vi "template-name.other.vi"(8 "error in (no error)":errorcluster, 10 "Numeric":dbl, 11 "class template-name in":refnum<class "template-name.lvclass">) -> (0 "error out":errorcluster, 2 "indicator template-name 2":dbl, 3 "class template-name out":refnum<class "template-name.lvclass">)   [LabVIEW 2019, in "template-name.lvclass"]
uses:
  template-name.lvclass
  template-name.control.ctl
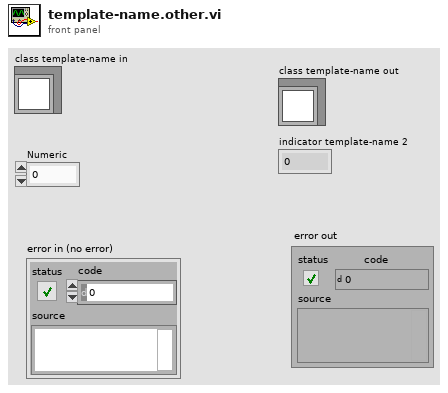
[diagram p1: front panel]
types:
  T1 = typedef "template-name.lvclass/template-name.control.ctl" = cluster{"Slide":dbl}
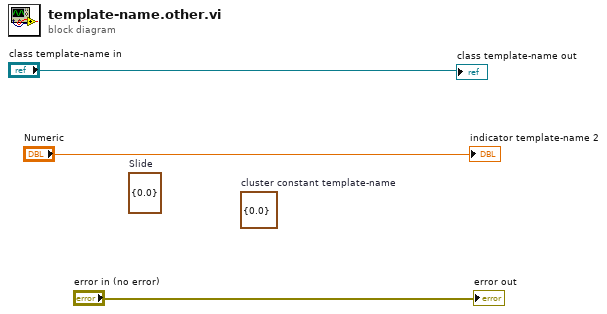
[diagram p0: block diagram]
diagram:
  (unwired) T1 {"Slide"=0.0}  # cluster constant template-name
  (unwired) T1 {"Slide"=0.0}  # Slide
  "class template-name out" <- "class template-name in"
  "indicator template-name 2" <- "Numeric"
  "error out" <- "error in (no error)"
